vi "Write udp receive session.vi"(8 "error in (no error)":errorcluster, 10 "udp receive session":refnum<k16>, 11 "UDP_receiver in":refnum<class "UDP_receiver.lvclass">) -> (0 "error out":errorcluster, 3 "UDP_receiver out":refnum<class "UDP_receiver.lvclass">)   [LabVIEW 2025, in "UDP_receiver.lvlib" / "UDP_receiver.lvclass"]
uses:
  UDP_receiver.lvclass
  UDP_receiver.lvclass/UDP_receiver.ctl
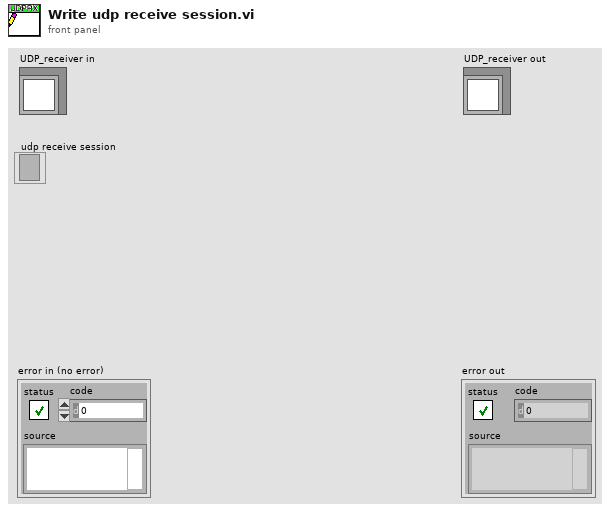
[diagram p1: front panel]
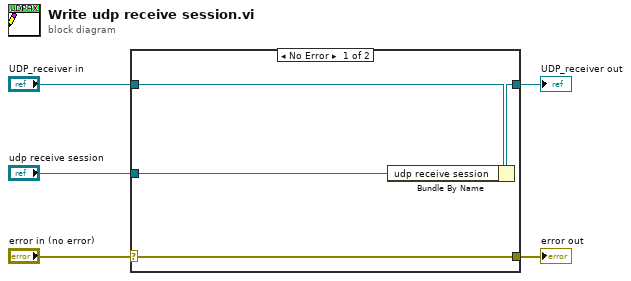
[diagram p0: block diagram]
diagram:
  n1 = case shown="No Error" "error in (no error)" {
    selector: "error in (no error)" -> [w9 w10]
    tunnel: [w9 w10] -> w4
    tunnel: [w7 w11] -> w2
    tunnel: "UDP_receiver in" -> [w8 w11]
    tunnel: "udp receive session" -> [w6 _]
    frame No Error {
      n2 = Bundle By Name(cluster=w8, "udp receive session"=w6) -> (w7:refnum<class "UDP_receiver.lvclass">)
    }
    frame Error {
    }
  }
  "error out" <- w4
  "UDP_receiver out" <- w2
